vi "Tester.vi"() -> ()   [LabVIEW 2020, in "Event Source.lvlib" / "Event Source Actor.lvclass"]
uses:
  Event Source Actor.lvclass
  Event Source Actor.lvclass/Event Source Actor.ctl
  <vilib>/ActorFramework/Message Queue/Message Queue.lvclass
  <vilib>/ActorFramework/Message Dequeuer/Message Dequeuer.lvclass
  Event Data/Event Data.lvclass
panel:
  out "Msg":string
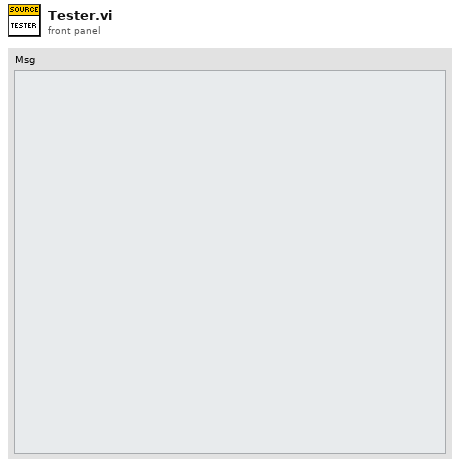
[diagram p1: front panel]
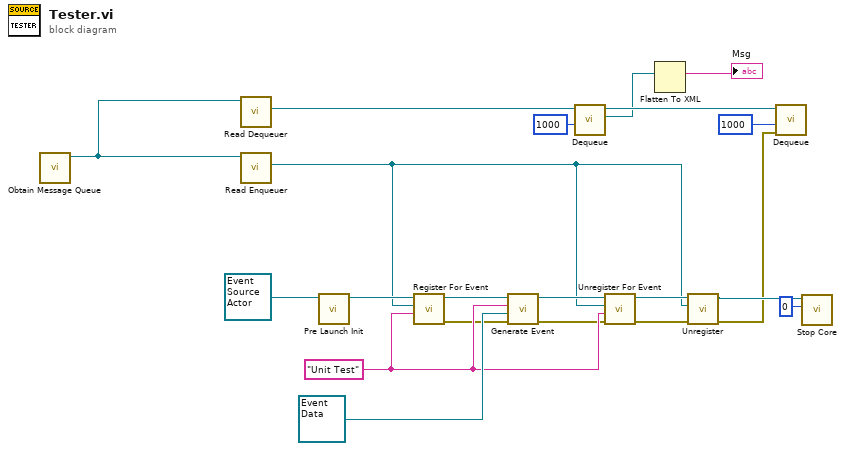
[diagram p0: block diagram]
diagram:
  w9 = "Unit Test" ("Event Name")
  n1 = call <vilib>:"Obtain Message Queue.vi"() -> ("Message Queue"=w21:refnum<class "Message Queue.lvclass">)  [unwired: 10 in, 1 out]
  n2 = call <vilib>:"Read Dequeuer.vi"("Message Queue"=w21) -> ("Message Dequeuer"=w20:refnum<class "Message Dequeuer.lvclass">)  [unwired: 10 in]
  n3 = call <vilib>:"Read Enqueuer.vi"("Message Queue"=w21) -> ("Message Enqueuer"=w5:refnum<class "Message Enqueuer.lvclass">)  [unwired: 10 in]
  n4 = call-dynamic "Pre Launch Init.vi"("Event Source In"=refnum<class "Event Source Actor.lvclass"> refnum ("Event Source.lvlib:Event Source.lvclass")) -> ("Event Source Out"=w14:refnum<class "Event Source Actor.lvclass">)  [unwired: 9 in, 1 out]
  n5 = call-dynamic "Register For Event.vi"("Event Name"=w9, "Registrant Enq"=w5, "Event Source Actor In"=w14) -> ("Error Out"=w3:errorcluster, "Event Source Actor Out"=w13:refnum<class "Event Source Actor.lvclass">)  [unwired: 7 in]
  n6 = call-dynamic "Generate Event.vi"("Error In"=w3, "Event Data"=refnum<class "Event Data.lvclass"> refnum, "Event Name"=w9, "Event Source In"=w13) -> ("Error Out"=w2:errorcluster, "Event Source Out"=w8:refnum<class "Event Source Actor.lvclass">)  [unwired: 6 in]
  n7 = call <vilib>:"Dequeue.vi"("timeout in ms (-1)"=1000, "Message Dequeuer in"=w20) -> ("Message"=w11:refnum<class "Message.lvclass">, "Message Dequeuer out"=w19:refnum<class "Message Dequeuer.lvclass">)  [unwired: 5 in, 3 out]
  n8 = call-dynamic "Unregister For Event.vi"("Error In"=w2, "Event Name"=w9, "Registrant Address"=w5, "Event Source Actor In"=w8) -> ("Error Out"=w1:errorcluster, "Event Source Actor Out"=w7:refnum<class "Event Source Actor.lvclass">)  [unwired: 6 in]
  n9 = Flatten To XML(6:w11) -> (2:→"Msg":string)
  n10 = call-dynamic "Unregister.vi"("Error In"=w1, "Registrant Enq"=w5, "Event Source In"=w7) -> ("Error Out"=w4:errorcluster, "Event Source Out"=w6:refnum<class "Event Source Actor.lvclass">)  [unwired: 7 in]
  n11 = call <vilib>:"Dequeue.vi"("error in (no error)"=w4, "timeout in ms (-1)"=1000, "Message Dequeuer in"=w19) -> ()  [unwired: 4 in, 5 out]
  n12 = call-dynamic "Stop Core.vi"("final error code"=0, "Event Source In"=w6) -> ()  [unwired: 9 in, 1 out]
